vi "Current VI Path.vi"(4 "error in":errorcluster, 6 "file name":string="open.txt", 7 "path":path) -> (0 "error out":errorcluster, 3 "Path for file":path)   [LabVIEW 2012]
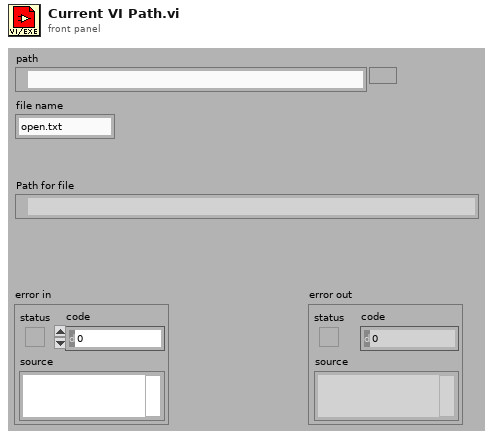
[diagram p1: front panel]
types:
  T1 = enum32{"invalid app kind", "Development System", "Run Time System", "Student Edition", "Embedded LabVIEW", "Evaluation", "Custom"}
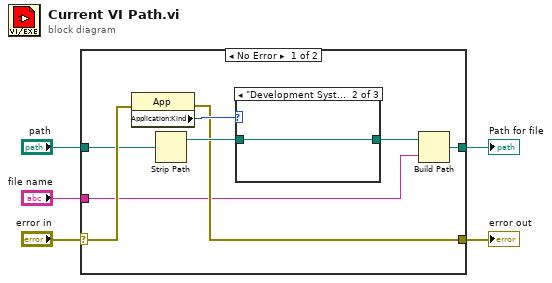
[diagram p0: block diagram]
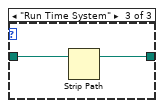
[diagram p3: hidden frame]
diagram:
  n1 = case shown="No Error" "error in" {
    selector: "error in" -> [w10 w18]
    tunnel: [w9 w18] -> w4
    tunnel: "path" -> [w8 w19]
    tunnel: [w7 w19] -> w2
    tunnel: "file name" -> [w6 _]
    frame No Error {
      n2 = property class="App"(error in=w10) -> (error out=w9:errorcluster, "Application:Kind"=w13:T1)  [unwired: 1 in, 1 out]
      n3 = Strip Path(path=w8) -> (stripped path=w11:path)  [unwired: 1 out]
      n4 = case shown="\"Development System\"" w13 {
        tunnel: [w14 w15 w17] -> w12
        tunnel: w11 -> [w14 w15 w16]
        frame Default {
        }
        frame "Development System" {
        }
        frame "Run Time System" {
          n5 = Strip Path(path=w16) -> (stripped path=w17:path)  [unwired: 1 out]
        }
      }
      n6 = Build Path(base path=w12, name or relative path=w6) -> (appended path=w7:path)
    }
    frame Error {
    }
  }
  "error out" <- w4
  "Path for file" <- w2
